vi "Pre Launch Init.vi"(11 "UI Controller in":refnum<class "UI Controller.lvclass">) -> (0 "error out":errorcluster, 3 "UI Controller out":refnum<class "UI Controller.lvclass">)   [LabVIEW 2019, in "UI Controller.lvlib" / "UI Controller.lvclass"]
doc: "(<B>Filename</B>: Actor Framework.lvlib:Actor.lvclass:Pre Launch Init.vi)\n\nDefines behavior that occurs after the Launch Nested Actor method is invoked but before the actor's Actor Core method begins running.\n\nBy default, this method does nothing. A descendant class may override it to define behavior."
uses:
  UI Controller.lvclass
  UI Controller.lvclass/UI Controller.ctl
  <vilib>/ActorFramework/Actor/Actor.lvclass
  UI Controller Messages/Update Event List Msg/Update Event List Msg.lvclass
  C:/Program Files (x86)/National Instruments/LabVIEW 2019/vi.lib/ActorFramework/Actor/Actor.lvclass
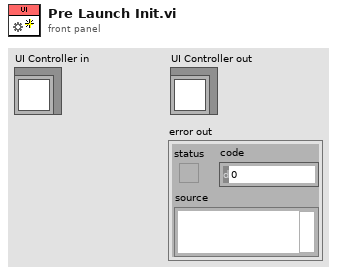
[diagram p1: front panel]
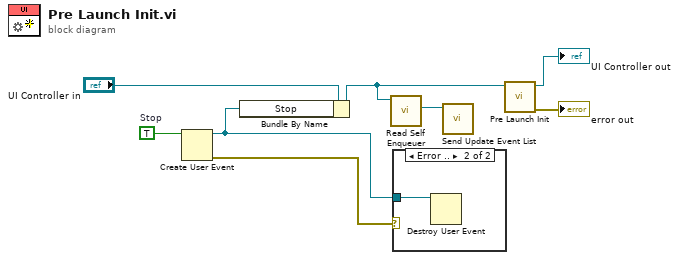
[diagram p0: block diagram]
diagram:
  w6 = TRUE  # Stop
  n1 = Create User Event(user event datatype=w6) -> (user event=w3:refnum<user-event>, error out=w4:errorcluster)  [unwired: 1 in]
  n2 = Bundle By Name(cluster="UI Controller in", "Stop"=w3) -> (w2:refnum<class "UI Controller.lvclass">)
  n3 = call <vilib>:"Read Self Enqueuer.vi"("Actor"=w2) -> ("Self Enqueuer"=w1:refnum<class "Message Enqueuer.lvclass">)  [unwired: 10 in]
  n4 = case shown="Error .." w4 {
    tunnel: w3 -> [_ w9]
    frame No Error {
    }
    frame Error {
      n5 = Destroy User Event(user event=w9) -> ()  [unwired: 1 in, 1 out]
    }
  }
  n6 = call "Send Update Event List.vi"("Message Enqueuer"=w1) -> ()  [unwired: 9 in, 2 out]
  n7 = call-parent "Pre Launch Init.vi"("Actor in"=w2) -> ("error out"=→"error out":errorcluster, "Actor out"=→"UI Controller out":refnum<class "UI Controller.lvclass">)  [unwired: 9 in]
